vi "Display and Save Single Shot Taus.vi"(8 "error in":errorcluster, 10 "state":T1, 11 "fileRefIn":refnum<file>) -> (0 "error out":errorcluster)   [LabVIEW 2012]
uses:
  tau_state.ctl
panel:
  out "time":timestamp format="%<%H:%M:%S%2u>T"
  out "tau":sgl[][](graph)
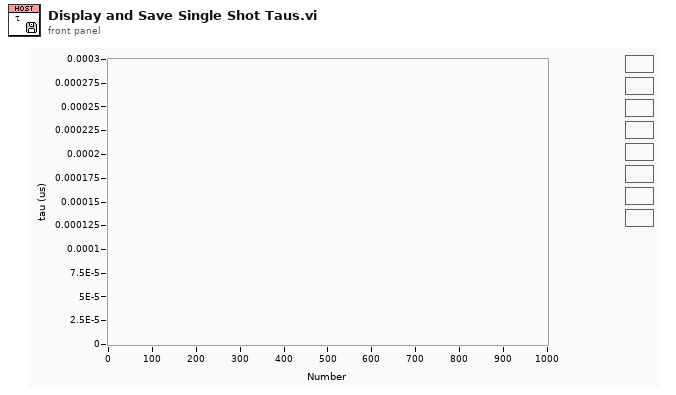
[diagram p1: front panel]
types:
  T1 = typedef "tau_state.ctl" = enum16{"Config", "Write", "Close"}
  T2 = enum16{"open", "replace", "create", "open or create", "replace or create", "replace or create with confirmation"}
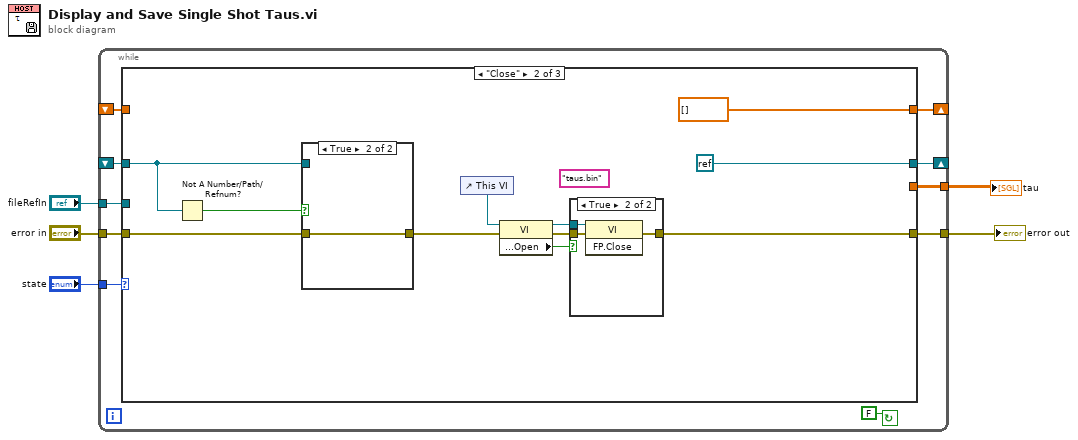
[diagram p0: block diagram]
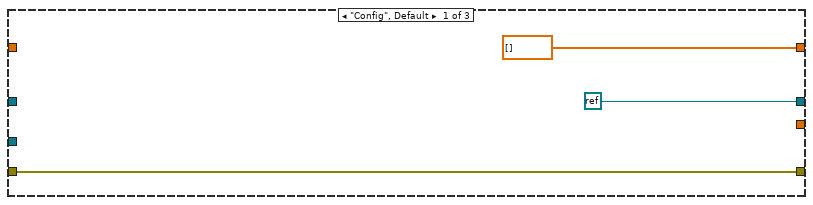
[diagram p2: hidden frame]
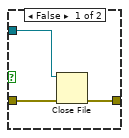
[diagram p3: hidden frame]
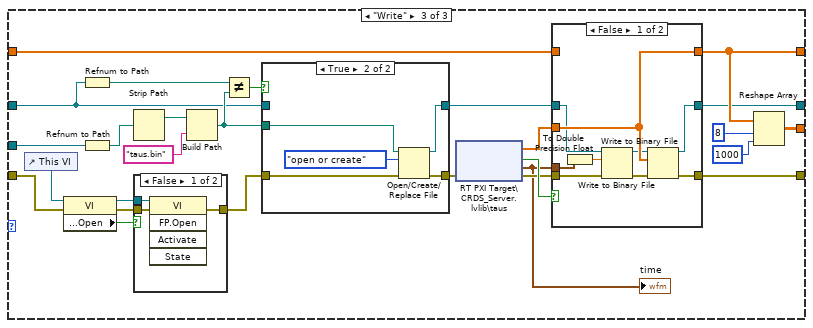
[diagram p5: hidden frame]
diagram:
  n1 = while {
    shift-right: [w8] -> _
    shift-left: _ -> [w9]
    tunnel: "error in" -> [w15]
    tunnel: [w11] -> w4
    tunnel: "fileRefIn" -> [w14]
    shift-right: [w12] -> _
    shift-left: _ -> [w13]
    tunnel: "state" -> [w7]
    tunnel: [w6] -> w1
    stop <- FALSE continue-if-true
    n2 = case shown="\"Close\"" w7 {
      tunnel: w15 -> [w16 w27 w40]
      tunnel: w14 -> [_ _ w59]
      tunnel: w13 -> [_ w20 w55]
      tunnel: [refnum<k0> refnum ("refnum out") refnum<k0> refnum ("refnum out") w49] -> w12
      tunnel: [w16 w21 w46] -> w11
      tunnel: w9 -> [_ _ w54]
      tunnel: [sgl[] [] ("Array of Single") sgl[] [] ("Array of Single") w51] -> w8
      tunnel: [_ _ w45] -> w6
      frame "Config", Default {
      }
      frame "Close" {
        (unwired) "taus.bin" ("name or relative path")
        n3 = Not A Number/Path/Refnum?(number/path/refnum=w20) -> (NaN/Path/Refnum?=w19:bool)
        n4 = case shown="True" w19 {
          tunnel: w27 -> [w32 w33]
          tunnel: [w31 w33] -> w22
          tunnel: w20 -> [w30 _]
          frame False {
            n5 = Close File(refnum=w30, error in=w32) -> (error out=w31:errorcluster)  [unwired: 1 out]
          }
          frame True {
          }
        }
        n6 = control-ref of="This VI"() -> (w26:refnum<vi>)
        n7 = property class="VI"(reference=w26, error in=w22) -> (reference out=w24:refnum<vi>, error out=w23:errorcluster, "Front Panel.Open"=w25:bool)
        n8 = case shown="True" w25 {
          tunnel: w24 -> [_ w37]
          tunnel: w23 -> [w34 w36]
          tunnel: [w34 w35] -> w21
          frame False {
          }
          frame True {
            n9 = invoke class="VI" method="FP.Close"(reference=w37, error in=w36) -> (error out=w35:errorcluster)  [unwired: 1 in, 2 out]
          }
        }
      }
      frame "Write" {
        n10 = control-ref of="This VI"() -> (w44:refnum<vi>)
        n11 = property class="VI"(reference=w44, error in=w40) -> (reference out=w42:refnum<vi>, error out=w41:errorcluster, "Front Panel.Open"=w43:bool)
        n12 = Refnum to Path(1:w55) -> (0:w58:path)
        n13 = Refnum to Path(1:w59) -> (0:w60:path)
        n14 = Strip Path(path=w60) -> (stripped path=w61:path)  [unwired: 1 out]
        n15 = case shown="False" w43 {
          tunnel: w42 -> [w67 _]
          tunnel: w41 -> [w66 w68]
          tunnel: [w65 w68] -> w39
          frame False {
            n16 = invoke class="VI" method="FP.Open"(reference=w67, error in=w66) -> (error out=w65:errorcluster)  [unwired: 3 in, 4 out]
          }
          frame True {
          }
        }
        n17 = Build Path(base path=w61, name or relative path="taus.bin") -> (appended path=w57:path)
        n18 = Not Equal?(x=w58, y=w57) -> (x != y?=w56:bool)
        n19 = case shown="True" w56 {
          tunnel: [w82 w87] -> w50
          tunnel: w55 -> [w82 _]
          tunnel: w57 -> [_ w85]
          tunnel: [w81 w84] -> w48
          tunnel: w39 -> [w81 w83]
          frame False {
          }
          frame True {
            n20 = Open/Create/Replace File(file path (use dialog)=w85, error in=w83, operation (0:open)=T2."open or create") -> (refnum out=w87:refnum<file>, error out=w84:errorcluster)  [unwired: 3 in, 1 out]
          }
        }
        n21 = shared-variable "RT PXI Target\\CRDS_Server.lvlib\\taus"(error in=w48) -> (w53:sgl[], error out=w47:errorcluster, w52:bool, w38:timestamp)  [unwired: 1 in]
        "time" <- w38
        n22 = case shown="False" w52 {
          tunnel: w53 -> [w77 _]
          tunnel: [w77 w80] -> w51
          tunnel: w54 -> [_ w80]
          tunnel: w50 -> [w74 w78]
          tunnel: [w76 w78] -> w49
          tunnel: w47 -> [w69 w79]
          tunnel: [w75 w79] -> w46
          tunnel: w38 -> [w71 _]
          frame False {
            n23 = To Double Precision Float(number=w71) -> (double precision float=w70:dbl)
            n24 = Write to Binary File(file (use dialog)=w74, data=w70, error in=w69) -> (refnum out=w73:refnum<file>, error out=w72:errorcluster)  [unwired: 3 in, 1 out]
            n25 = Write to Binary File(file (use dialog)=w73, data=w77, error in=w72) -> (refnum out=w76:refnum<file>, error out=w75:errorcluster)  [unwired: 3 in, 1 out]
          }
          frame True {
          }
        }
        n26 = Reshape Array(w51, 8 ("dimension size"), 1000 ("dimension size")) -> (w45:sgl[][])
      }
    }
  }
  "error out" <- w4
  "tau" <- w1
